vi "REPLACE.vi"(7 "Actor in":refnum<class "Actor.lvclass">, 11 "State in":refnum<class "State.lvclass">) -> (2 "Destroy?":bool, 5 "Actor out":refnum<class "Actor.lvclass">)   [LabVIEW 2021, in "jettl.lvlib" / "State.lvclass"]
uses:
  State.lvclass
  Actor/Actor/Actor.lvclass
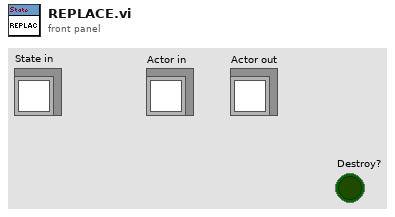
[diagram p1: front panel]
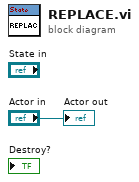
[diagram p0: block diagram]
diagram:
  "Actor out" <- "Actor in"
